vi "Get Virtual Folder if Exists.vi"(8 "error in (no error)":errorcluster, 9 "Virtual Folder Name":string, 11 "LVClassLibrary Refnum in":refnum<vi>) -> (0 "error out":errorcluster, 1 "Folder Refnum out":refnum<vi>, 3 "LVClassLibrary Refnum out":refnum<vi>)   [LabVIEW 2021, in "MemberVICreation.lvlib" / "BaseAccessorScripter.lvclass"]
uses:
  <resource>/Framework/Providers/LVClassLibrary/NewAccessors/BaseAccessorScripter/BaseAccessorScripter.lvclass
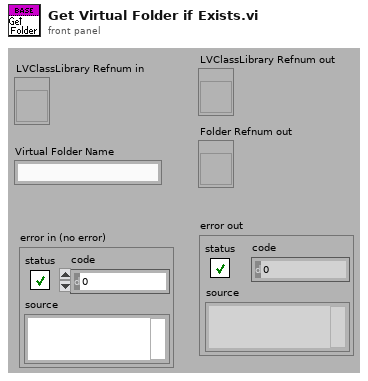
[diagram p1: front panel]
types:
  T1 = typedef "LIBUIP_item_type.ctl" = enum16{"None", "ParentLib", "Property Def Item", "VI", "Non-VI", "Folder", "Library", "Menu", "XI Ability VI", "XI Method VI", "XI Property VI", "Property Folder", "Class Private Data"}
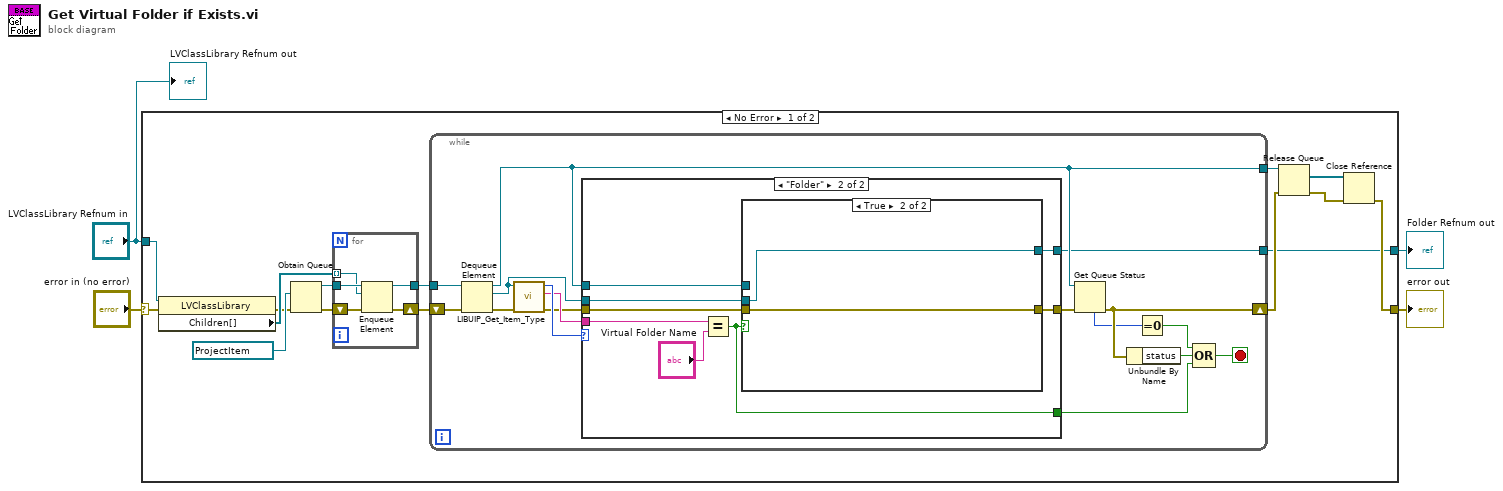
[diagram p0: block diagram]
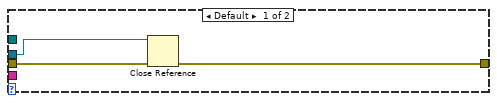
[diagram p2: hidden frame]
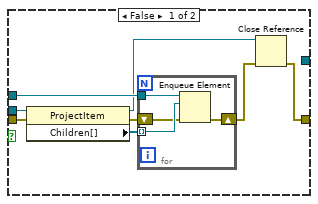
[diagram p3: hidden frame]
diagram:
  n1 = case shown="No Error" "error in (no error)" {
    selector: "error in (no error)" -> [w5 w66]
    tunnel: [w7 w66] -> w3
    tunnel: "LVClassLibrary Refnum in" -> [w19 _]
    tunnel: [w6 _] -> w1
    frame No Error {
      n2 = property class="LVClassLibrary"(reference=w19, error in=w5) -> (error out=w12:errorcluster, "Children[]"=w18:refnum<vi>[])  [unwired: 1 out]
      n3 = Obtain Queue(element data type=refnum<vi> refnum ("ProjectItem Refnum"), error in (no error)=w12) -> (queue out=w16:refnum<queue>, error out=w15:errorcluster)  [unwired: 2 in, 2 out]
      n4 = for {
        tunnel: w18 -> [w23] mode=indexing
        tunnel: w16 -> [w24]
        tunnel: [w20] -> w14
        shift-right: [w21] -> w13
        shift-left: w15 -> [w22]
        n5 = Enqueue Element(queue=w24, element=w23, error in (no error)=w22) -> (queue out=w20:refnum<queue>, error out=w21:errorcluster)  [unwired: 2 out]
      }
      n6 = while {
        tunnel: w14 -> [w39]
        shift-right: [w29] -> w8
        shift-left: w13 -> [w40]
        tunnel: [w26] -> w11
        tunnel: [w25] -> w6
        stop <- w35 stop-if-true
        n7 = Dequeue Element(queue=w39, error in (no error)=w40) -> (queue out=w26:refnum<queue>, element=w38:refnum<vi>, error out=w37:errorcluster)  [unwired: 2 out]
        n8 = call <resource>:"LIBUIP_Get_Item_Type.vi"("error in (no error)"=w37, "ProjectItem Refnum"=w38) -> ("error out"=w31:errorcluster, "Name"=w32:string, "Type"=w33:T1)  [unwired: 7 out]
        n9 = case shown="\"Folder\"" w33 {
          tunnel: [_ w49] -> w36
          tunnel: w32 -> [_ w50]
          tunnel: w38 -> [w43 w48]
          tunnel: w26 -> [_ w47]
          tunnel: w31 -> [w42 w46]
          tunnel: [w41 w45] -> w30
          tunnel: [_ w44] -> w25
          frame Default {
            n10 = Close Reference(reference=w43, error in (no error)=w42) -> (error out=w41:errorcluster)
          }
          frame "Folder" {
            n11 = Equal?(x=w50, y="Virtual Folder Name") -> (x = y?=w49:bool)
            n12 = case shown="True" w49 {
              tunnel: w48 -> [w59 w64]
              tunnel: w47 -> [w57 _]
              tunnel: w46 -> [w56 w65]
              tunnel: [w52 w65] -> w45
              tunnel: [_ w64] -> w44
              frame False {
                n13 = property class="ProjectItem"(reference=w59, error in=w56) -> (reference out=w54:refnum<vi>, error out=w55:errorcluster, "Children[]"=w58:refnum<vi>[])
                n14 = for {
                  tunnel: w58 -> [w63] mode=indexing
                  tunnel: w57 -> [w62]
                  shift-right: [w60] -> w53
                  shift-left: w55 -> [w61]
                  n15 = Enqueue Element(queue=w62, element=w63, error in (no error)=w61) -> (error out=w60:errorcluster)  [unwired: 3 out]
                }
                n16 = Close Reference(reference=w54, error in (no error)=w53) -> (error out=w52:errorcluster)
              }
              frame True {
              }
            }
          }
        }
        n17 = Get Queue Status(queue=w26, error in (no error)=w30) -> (error out=w29:errorcluster, # elements in queue=w28:i32)  [unwired: 7 out]
        n18 = Unbundle By Name(w29) -> ("status"=w34:bool)
        n19 = Equal To 0?(x=w28) -> (x = 0?=w27:bool)
        n20 = Compound Arithmetic op=OR(w27, w34, w36) -> (w35:bool)
      }
      n21 = Release Queue(queue=w11, error in (no error)=w8) -> (remaining elements=w10:refnum<vi>[], error out=w9:errorcluster)  [unwired: 2 out]
      n22 = Close Reference(reference=w10, error in (no error)=w9) -> (error out=w7:errorcluster)
    }
    frame Error {
    }
  }
  "error out" <- w3
  "Folder Refnum out" <- w1
  "LVClassLibrary Refnum out" <- "LVClassLibrary Refnum in"
